vi "ReadDynamixelInformation.vi"(8 "error in (no error)":errorcluster, 9 "VISA resource name":refnum<visa-resource-name>, 10 "DynamixelTorque Queue":refnum<queue>, 11 "Notifier References":T1) -> (0 "error out":errorcluster, 3 "Load/Torque Array":dbl[](array[numeric]))   [LabVIEW 2013]
doc: "Reads Dynamixel torque off of the indicated Dynamixel and writes it to a queue.\n\nEric Schneider, March 2014"
uses:
  Data/TypeDefs/Notifiers.ctl
  Data/TypeDefs/UTM Location.ctl
  Data/TypeDefs/Sail Set Suggestions.ctl
  Data/TypeDefs/Rudder Set Suggestions.ctl
  Data/TypeDefs/OverrideInformation.ctl
  Data/TypeDefs/OverrideMode.ctl
  Data/TypeDefs/MotorSetup.ctl
  Data/TypeDefs/DynamixelSetupInfo.ctl
  Data/TypeDefs/AirmarStatus.ctl
  Data/TypeDefs/HardwareOnline.ctl
  Data/TypeDefs/DynamixelCycleTracker.ctl
  Data/TypeDefs/RC Input Values.ctl
  Classes/Waypoint/Waypoint.lvclass
  <instrlib>/Dynamixel Motor/Dynamixel Motor.lvlib
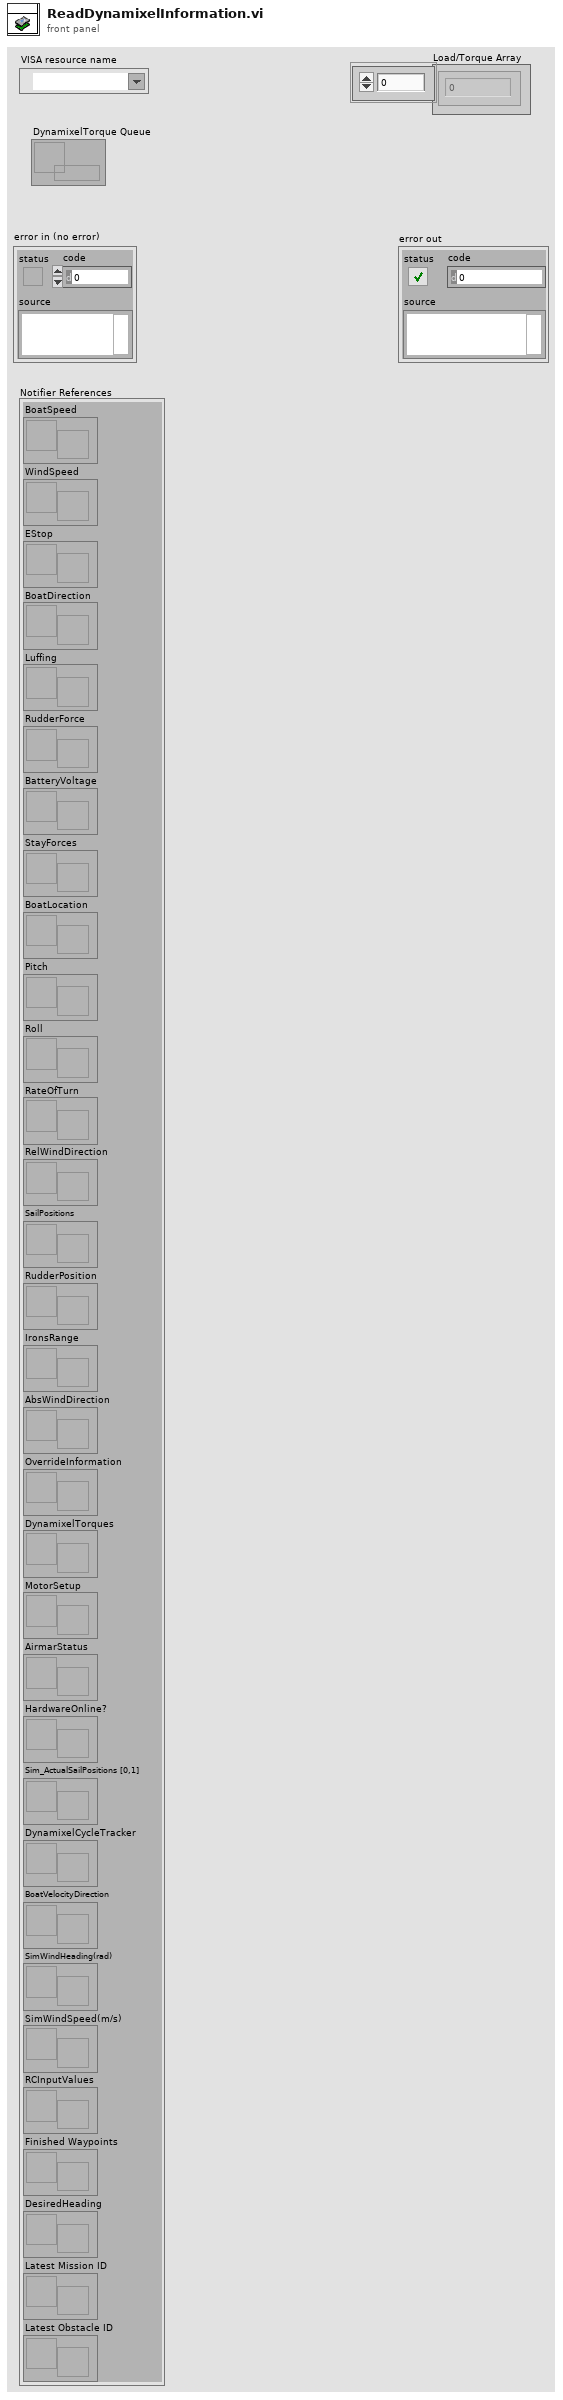
[diagram p1: front panel]
types:
  T1 = typedef "Notifiers.ctl" = cluster{"BoatSpeed":refnum<notifier>, "WindSpeed":refnum<notifier>, "EStop":refnum<notifier>, "BoatDirection":refnum<notifier>, "Luffing":refnum<notifier>, "RudderForce":refnum<notifier>, "BatteryVoltage":refnum<notifier>, "StayForces":refnum<notifier>, "BoatLocation":refnum<notifier>, "Pitch":refnum<notifier>, "Roll":refnum<notifier>, "RateOfTurn":refnum<notifier>, "RelWindDirection":refnum<notifier>, "SailPositions":refnum<notifier>, "RudderPosition":refnum<notifier>, "IronsRange":refnum<notifier>, "AbsWindDirection":refnum<notifier>, "OverrideInformation":refnum<notifier>, "DynamixelTorques":refnum<notifier>, "MotorSetup":refnum<notifier>, "AirmarStatus":refnum<notifier>, "HardwareOnline?":refnum<notifier>, "Sim_ActualSailPositions [0,1]":refnum<notifier>, "DynamixelCycleTracker":refnum<notifier>, "BoatVelocityDirection":refnum<notifier>, "SimWindHeading(rad)":refnum<notifier>, "SimWindSpeed(m/s)":refnum<notifier>, "RCInputValues":refnum<notifier>, "Finished Waypoints":refnum<notifier>, "DesiredHeading":refnum<notifier>, "Latest Mission ID":refnum<notifier>, "Latest Obstacle ID":refnum<notifier>}
  T2 = typedef "HardwareOnline.ctl" = cluster{"AirmarOnline":bool, "WindvaneOnline":bool, "HemisphereOnline":bool, "StayForceOnline":bool, "BatteryVoltageOnline":bool, "AccelerometerOnline":bool, "MainDynamixel Online":bool, "JibDynamixel Online":bool, "RudderDynamixel Online":bool}
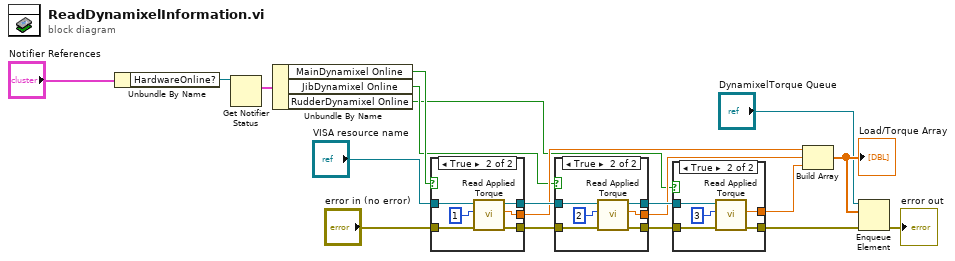
[diagram p0: block diagram]
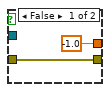
[diagram p2: hidden frame]
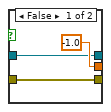
[diagram p3: hidden frame]
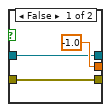
[diagram p4: hidden frame]
diagram:
  n1 = Unbundle By Name("Notifier References") -> ("HardwareOnline?"=w9:refnum<notifier>)
  n2 = Get Notifier Status(notifier=w9) -> (current notification=w8:T2)  [unwired: 1 in, 4 out]
  n3 = Unbundle By Name(w8) -> ("MainDynamixel Online"=w7:bool, "JibDynamixel Online"=w6:bool, "RudderDynamixel Online"=w5:bool)
  n4 = case shown="True" w7 {
    tunnel: "VISA resource name" -> [w21 w24]
    tunnel: "error in (no error)" -> [w20 w25]
    tunnel: [w21 w27] -> w19
    tunnel: [w20 w26] -> w18
    tunnel: [-1.0 ("Position (deg)") w28] -> w15
    frame False {
    }
    frame True {
      n5 = call <instrlib>:"Read Applied Torque.vi"("error in (no error)"=w25, "Motor ID (0)"=u8 1, "VISA resource name"=w24) -> ("error out"=w26:errorcluster, "Load/torque %"=w28:sgl, "VISA resource name out"=w27:refnum<visa-resource-name>)  [unwired: 6 in]
    }
  }
  n6 = case shown="True" w6 {
    tunnel: w19 -> [w29 w37]
    tunnel: w18 -> [w30 w36]
    tunnel: [w29 w34] -> w17
    tunnel: [w30 w32] -> w16
    tunnel: [-1.0 ("Position (deg)") w33] -> w14
    frame False {
    }
    frame True {
      n7 = call <instrlib>:"Read Applied Torque.vi"("error in (no error)"=w36, "Motor ID (0)"=u8 2, "VISA resource name"=w37) -> ("error out"=w32:errorcluster, "Load/torque %"=w33:sgl, "VISA resource name out"=w34:refnum<visa-resource-name>)  [unwired: 6 in]
    }
  }
  n8 = case shown="True" w5 {
    tunnel: w17 -> [_ w41]
    tunnel: w16 -> [w38 w42]
    tunnel: [-1.0 ("Position (deg)") w44] -> w13
    tunnel: [w38 w43] -> w12
    frame False {
    }
    frame True {
      n9 = call <instrlib>:"Read Applied Torque.vi"("error in (no error)"=w42, "Motor ID (0)"=u8 3, "VISA resource name"=w41) -> ("error out"=w43:errorcluster, "Load/torque %"=w44:sgl)  [unwired: 6 in, 1 out]
    }
  }
  n10 = Build Array(w15, w14, w13) -> (w11:dbl[])
  "Load/Torque Array" <- w11
  n11 = Enqueue Element(queue="DynamixelTorque Queue", element=w11, error in (no error)=w12) -> (error out=→"error out":errorcluster)  [unwired: 1 in, 2 out]
